vi "sub_SDR_rx_PacketSynch.vi"(10 "Input Stream":string) -> (1 "Last received packet num":i32, 2 "Output Packets":string[](array[string]))   [LabVIEW 2012]
uses:
  <vilib>/imath/engines/lvmath/Plug In/_Char/NIMS_CH_character datatype.ctl
  <vilib>/imath/engines/lvmath2/RunTimeEngine/ErrorHandling/NIMS_Finalize Error.vi
  <vilib>/imath/engines/lvmath/Plug In/_Char/NIMS_CH_String to Character Array.vi
  <vilib>/imath/engines/lvmath2/RunTimeEngine/NodeEndStatement/NIMS_NodeEndStatement_Get Vector.vi
  <instcachedir>/0/NIMS_NodeEndStatement_Get Vector_2BE3967F82A04EDB90B65AFAEF9E88C9.lvgen/NIMS_NodeEndStatement_Get Vector_2BE3967F82A04EDB90B65AFAEF9E88C9_000.vi
  <vilib>/imath/engines/lvmath/Plug In/_Char/NIMS_CH_Character RV to String.vi
  <vilib>/imath/engines/lvmath2/RunTimeEngine/VariableToken/NIMS_VariableToken_CondDefined.vi
  <instcachedir>/0/NIMS_VariableToken_CondDefined_295AAB8C64C949DA8EA45AB7820AF759.lvgen/NIMS_VariableToken_CondDefined_295AAB8C64C949DA8EA45AB7820AF759_003.vi
  <vilib>/imathl/engines/lvmath/Functions/Error Handling/Create Error.vi
  <vilib>/imath/engines/lvmath/Functions/Error Handling/MergeErrorsWrapper.vi
  <vilib>/imath/engines/lvmath2/RunTimeEngine/NodeEndStatement/NIMS_NodeEndStatement_Output.vi
  <instcachedir>/0/NIMS_NodeEndStatement_Output_53EC0D466D134D7ABD903AC30B43404B.lvgen/NIMS_NodeEndStatement_Output_53EC0D466D134D7ABD903AC30B43404B_009.vi
  <vilib>/imath/engines/lvmath/Plug In/_Char/NIMS_CH_Character 2D to String 1D.vi
  <vilib>/imath/engines/lvmath2/RunTimeEngine/BuiltInFunctions/strconcat/NIMS_strconcat.vi
  <vilib>/imath/engines/lvmath/Plug In/_Char/NIMS_CH_String CV to Character 2D.vi
  <instcachedir>/0/NIMS_CH_String CV to Character 2D_B2E5264245B74746A343EBB64433A4F6.lvgen/NIMS_CH_String CV to Character 2D_B2E5264245B74746A343EBB64433A4F6_000.vi
  <vilib>/imath/engines/lvmath2/RunTimeSupport/NIMS_Get Row Vector_w Error - Matrix.vi
  <instcachedir>/0/NIMS_Get Row Vector_w Error - Matrix_6B6275C45A6E4FE79E77FBB7DADD2796.lvgen/NIMS_Get Row Vector_w Error - Matrix_6B6275C45A6E4FE79E77FBB7DADD2796_000.vi
  <vilib>/imath/engines/lvmath2/RunTimeEngine/BuiltInFunctions/findstr/NIMS_findstr.vi
  <vilib>/imath/engines/lvmath2/RunTimeEngine/BuiltInFunctions/length/NIMS_length(GV).vi
  <instcachedir>/0/NIMS_length(GV)_08A3D13377FD4E4B96F5795FBF3698FA.lvgen/NIMS_length(GV)_08A3D13377FD4E4B96F5795FBF3698FA_002.vi
  <vilib>/imath/engines/lvmath2/RunTimeEngine/BuiltInFunctions/length/NIMS_length(GM).vi
  <instcachedir>/0/NIMS_length(GM)_47CEC356FCE0482D9BA47DC61C99F2C7.lvgen/NIMS_length(GM)_47CEC356FCE0482D9BA47DC61C99F2C7_003.vi
  <vilib>/imath/engines/lvmath2/RunTimeEngine/VariableToken/Read/NIMS_Get Elements - SorM(_) - Check.vi
  <instcachedir>/0/NIMS_Get Elements - SorM(_) - Check_8FDA2664A675493882C25203DD903B51.lvgen/NIMS_Get Elements - SorM(_) - Check_8FDA2664A675493882C25203DD903B51_007.vi
  <vilib>/imath/engines/lvmath2/RunTimeEngine/VariableToken/Read/NIMS_Get Elements - RV(_) - Check.vi
  <instcachedir>/0/NIMS_Get Elements - RV(_) - Check_09E565EE58C54071A799578B82C9999A.lvgen/NIMS_Get Elements - RV(_) - Check_09E565EE58C54071A799578B82C9999A_003.vi
  <vilib>/imath/engines/lvmath2/RunTimeEngine/RangeToken/NIMS_Range_R2.vi
  <instcachedir>/0/NIMS_Get Elements - SorM(_) - Check_8FDA2664A675493882C25203DD903B51.lvgen/NIMS_Get Elements - SorM(_) - Check_8FDA2664A675493882C25203DD903B51_008.vi
  <vilib>/imath/engines/lvmath2/RunTimeEngine/ErrorHandling/NIMS_Create Error From Enums.vi
panel:
  out "Received Packets":i32
  out "CRC Fails":i32
  out "Internal Buffer":string
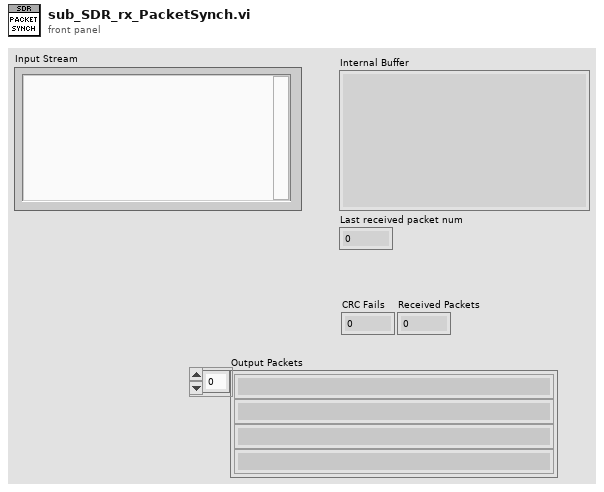
[diagram p1: front panel]
types:
  T1 = typedef "NIMS_CH_character datatype.ctl" = cluster{"Numeric":u8}
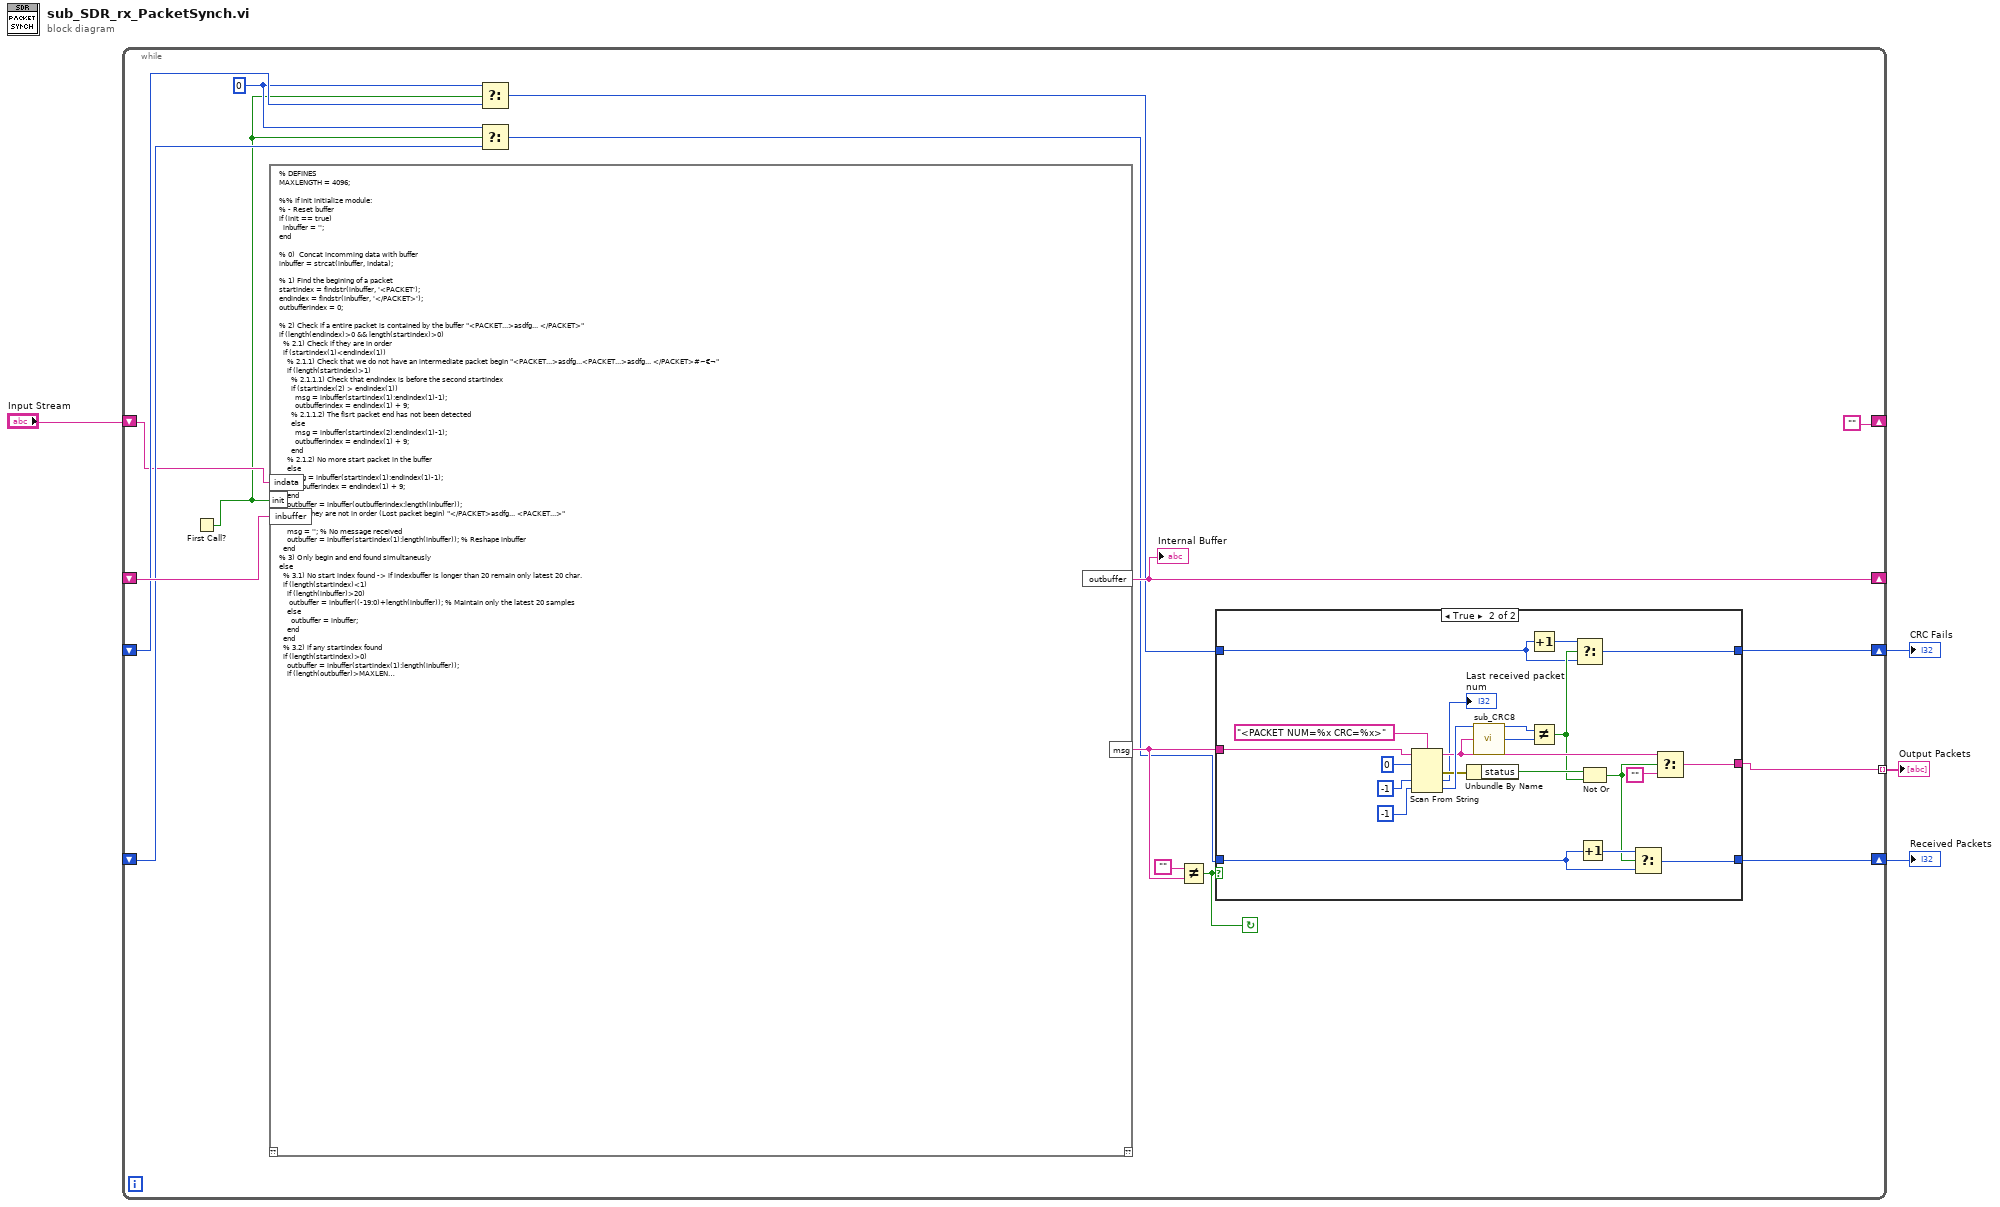
[diagram p0: block diagram]
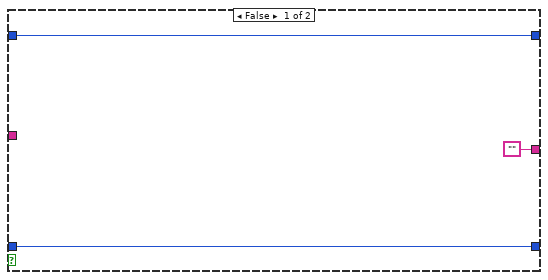
[diagram p2: hidden frame]
diagram:
  n1 = while {
    shift-right: [w20] -> _
    shift-left: _ -> [w19]
    shift-right: [w15] -> w4
    shift-left: _ -> [w16]
    shift-right: [w10] -> w3
    shift-left: _ -> [w11]
    tunnel: [w9] -> w2 mode=indexing
    shift-right: [""] -> _
    shift-left: "Input Stream" -> [w7]
    stop <- w8 continue-if-true
    w13 = 0 ("t")
    n2 = First Call?() -> (First Call?: T/F=w5:bool)
    n3 = mathscript code="% DEFINES\nMAXLENGTH = 4096;\n\n%% If init initialize module:\n% - Reset buffer\nif (init == true)\n  inbuffer = '';\nend\n\n% 0)  Concat incomming data with buffer\ninbuffer = strcat(inbuffer, indata);\n\n% 1) Find the begining of a packet\nstartindex = findstr(inbuffer, '<PACKET');\nendindex = findstr(inbuffer, '</PACKET>');\noutbufferindex = 0;\n\n% 2) Check if a entire packet is contained by the buffer \"<PACKET...>asdfg... </PACKET>\"\nif (length(endindex)>0 && length(startindex)>0)\n  % 2.1) Check if they are in order\n  if (startindex(1)<endindex(1))\n    % 2.1.1) Check that we do not have an intermediate packet begin \"<PACKET...>asdfg...<PACKET...>asdfg... </PACKET>#~€¬\"\n    if (length(startindex)>1)\n      % 2.1.1.1) Check that endindex is before the second startindex\n      if (startindex(2) > endindex(1))\n        msg = inbuffer(startindex(1):endindex(1)-1);\n        outbufferindex = endindex(1) + 9;\n      % 2.1.1.2) The fisrt packet end has not been detected\n      else\n        msg = inbuffer(startindex(2):endindex(1)-1); \n        outbufferindex = endindex(1) + 9;\n      end\n    % 2.1.2) No more start packet in the buffer\n    else\n      msg = inbuffer(startindex(1):endindex(1)-1);\n      outbufferindex = endindex(1) + 9;        \n    end\n    outbuffer = inbuffer(outbufferindex:length(inbuffer));\n  % 2.2) They are not in order (Lost packet begin) \"</PACKET>asdfg... <PACKET...>\"\n  else\n    msg = ''; % No message received\n    outbuffer = inbuffer(startindex(1):length(inbuffer)); % Reshape inbuffer\n  end\n% 3) Only begin and end found simultaneusly\nelse\n  % 3.1) No start index found -> if indexbuffer is longer than 20 remain only latest 20 char.\n  if (length(startindex)<1)\n    if (length(inbuffer)>20)\n     outbuffer = inbuffer((-19:0)+length(inbuffer)); % Maintain only the latest 20 samples\n    else\n      outbuffer = inbuffer;\n    end\n  end\n  % 3.2) if any startindex found\n  if (length(startindex)>0)\n    outbuffer = inbuffer(startindex(1):length(inbuffer));\n    if (length(outbuffer)>MAXLENGTH)\n        outbuffer = outbuffer ((length(outbuffer)-20):length(outbuffer));\n    end\n  end\n  msg = ''; % No message received\nend"("inbuffer"=w19, "indata"=w7, "init"=w5) -> ("outbuffer"=w20:string, "msg"=w17:string)  [unwired: 1 in, 1 out]
    "Internal Buffer" <- w20
    n4 = Select(t=w13, s=w5, f=w16) -> (s? t:f=w14:i32)
    n5 = Select(t=w13, s=w5, f=w11) -> (s? t:f=w12:i32)
    n6 = Not Equal?(x="", y=w17) -> (x != y?=w8:bool)
    n7 = case shown="True" w8 {
      tunnel: w17 -> [_ w39]
      tunnel: ["" w32] -> w9
      tunnel: [w22 w31] -> w15
      tunnel: w14 -> [w22 w28]
      tunnel: w12 -> [w21 w26]
      tunnel: [w21 w25] -> w10
      frame False {
      }
      frame True {
        n8 = Scan From String(format string="<PACKET NUM=%x CRC=%x>", input string=w39, initial scan location=u32 0, default 1=-1 ("default value 1"), default 2=-1 ("default value 2")) -> (remaining string=w35:string, error out=w38:errorcluster, output 1=→"Last received packet num":i32, output 2=w40:i32)  [unwired: 1 in, 1 out]
        n9 = Unbundle By Name(w38) -> ("status"=w37:bool)
        n10 = call "sub_CRC8.vi"("message"=w35) -> ("CRC8"=w41:u8)  [unwired: 4 in]
        n11 = Increment(x=w28) -> (x+1=w29:i32)
        n12 = Not Equal?(x=w40, y=w41) -> (x != y?=w30:bool)
        n13 = Select(t=w29, s=w30, f=w28) -> (s? t:f=w31:i32)
        n14 = Increment(x=w26) -> (x+1=w27:i32)
        n15 = Not Or(1:w30, 2:w37) -> (0:w24:bool)
        n16 = Select(t=w27, s=w24, f=w26) -> (s? t:f=w25:i32)
        n17 = Select(t=w35, s=w24, f="") -> (s? t:f=w32:string)
      }
    }
  }
  "CRC Fails" <- w4
  "Received Packets" <- w3
  "Output Packets" <- w2
